vi "robotoutputs.vi"() -> ()   [LabVIEW 2020]
doc: "This global variable contains current robot state information and actuator setpoints."
panel:
  out "Master_Caution":bool
  out "Number_of_Master_Alarms":i32
  out "Master_Alarm":bool
  out "Master_State":enum16{"Normal", "Climb"}(ring)
  out "LimeLight_PiP_Mode":T1(ring)
  out "Orientation Mode":T2(ring)
  out "Diverting_Power_LimeLight":bool
  out "LimeLight_Pipeline_Commanded":T3(ring)
  out "Current_Driver_Profile_Setpoints":dbl[](array[numeric])
  out "LED_Colors":u32[](array[colorbox])
  out "LimeLight_LED_Mode":enum16{"Pipeline Setting", "Off", "Blink", "On"}(ring)=enum."Off"
  out "Force_Low_Gear":bool
  out "Swerve_2_High_Gear_Requested":bool
  out "Swerve_1_High_Gear_Requested":bool
  out "Swerve_3_High_Gear_Requested":bool
  out "Swerve_0_High_Gear_Requested":bool
  out "Swerve_2_Drive_Flip":bool
  out "Swerve_1_Drive_Flip":bool
  out "Swerve_3_Drive_Flip":bool
  out "Swerve_0_Drive_Flip":bool
  out "Swerve_3_Azimuth_Goal (deg)":dbl
  out "Swerve_1_Azimuth_Goal (deg)":dbl
  out "Swerve_2_Azimuth_Goal (deg)":dbl
  out "Swerve_0_Azimuth_Goal (deg)":dbl
  out "Diverting_Power_LEDS":bool
  out "Swerve_Rotation_Command":dbl
  out "Disallowed_Master_States":bool[](array[boolean])
  out "Drive_Mode":enum16{"Driver Control", "Lock Heading"}(ring)
  out "Diverting_Power_Compressor":bool
  out "Confirmed_Master_States":bool[](array[boolean])
  out "Boost_Drive_Train":bool
  out "Swerve_3_Azimuth_Error (deg)":dbl
  out "Swerve_1_Azimuth_Error (deg)":dbl
  out "Swerve_2_Azimuth_Error (deg)":dbl
  out "Swerve_0_Azimuth_Error (deg)":dbl
  out "Swerve_3_Drive_Command":dbl
  out "Swerve_1_Drive_Command":dbl
  out "Swerve_2_Drive_Command":dbl
  out "Swerve_0_Drive_Command":dbl
  # "--power management--"
  # "--LL control--"
  # "--LEDs--"
  # "--master state controller--"
  # "--drivebase subsystem--"
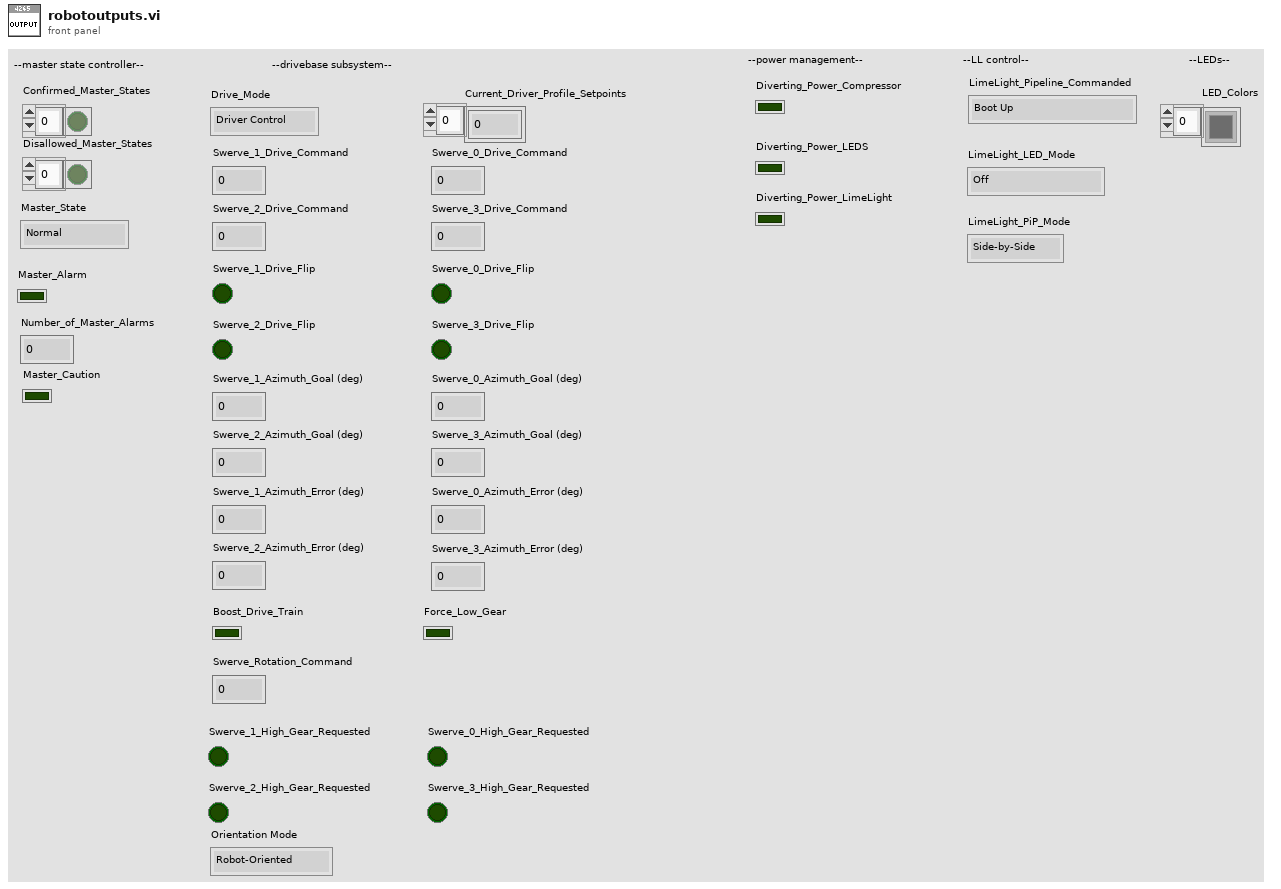
[diagram p1: front panel]
types:
  T1 = enum16{"Side-by-Side", "PiP Main", "PiP Secondary"}
  T2 = enum16{"Robot-Oriented", "Field-Oriented", "Intake"}
  T3 = enum16{"Boot Up", "Camera Override", "HUB Targeting", "CARGO Tracking"}
diagram:
